vi "CAN FD.vi"() -> ()   [LabVIEW 2018]
uses:
  <vilib>/xnet/xnet.llb/XNET Create Session (Signal Input Single-point).vi
  <vilib>/xnet/xnet.llb/XNET Read (Signal Single-point).vi
  <resource>/objmgr/xnet.rc
panel:
  out "CAN:FD ISO Mode":u32(ring) items=["ISO", "Non ISO", "ISO Legacy"]
  out "PDUs Required?":bool
  out "element":refnum<k21>
  in  "stop":bool
  out "data":dbl[](array[numeric]) format="%.2f"
  out "session out 2":refnum<k21>
  out "Signals":refnum<k21>[](array[refnum])
  in  "error in (no error)":errorcluster
  in  "DBC File Selection":refnum<k21>="CAN DATA"
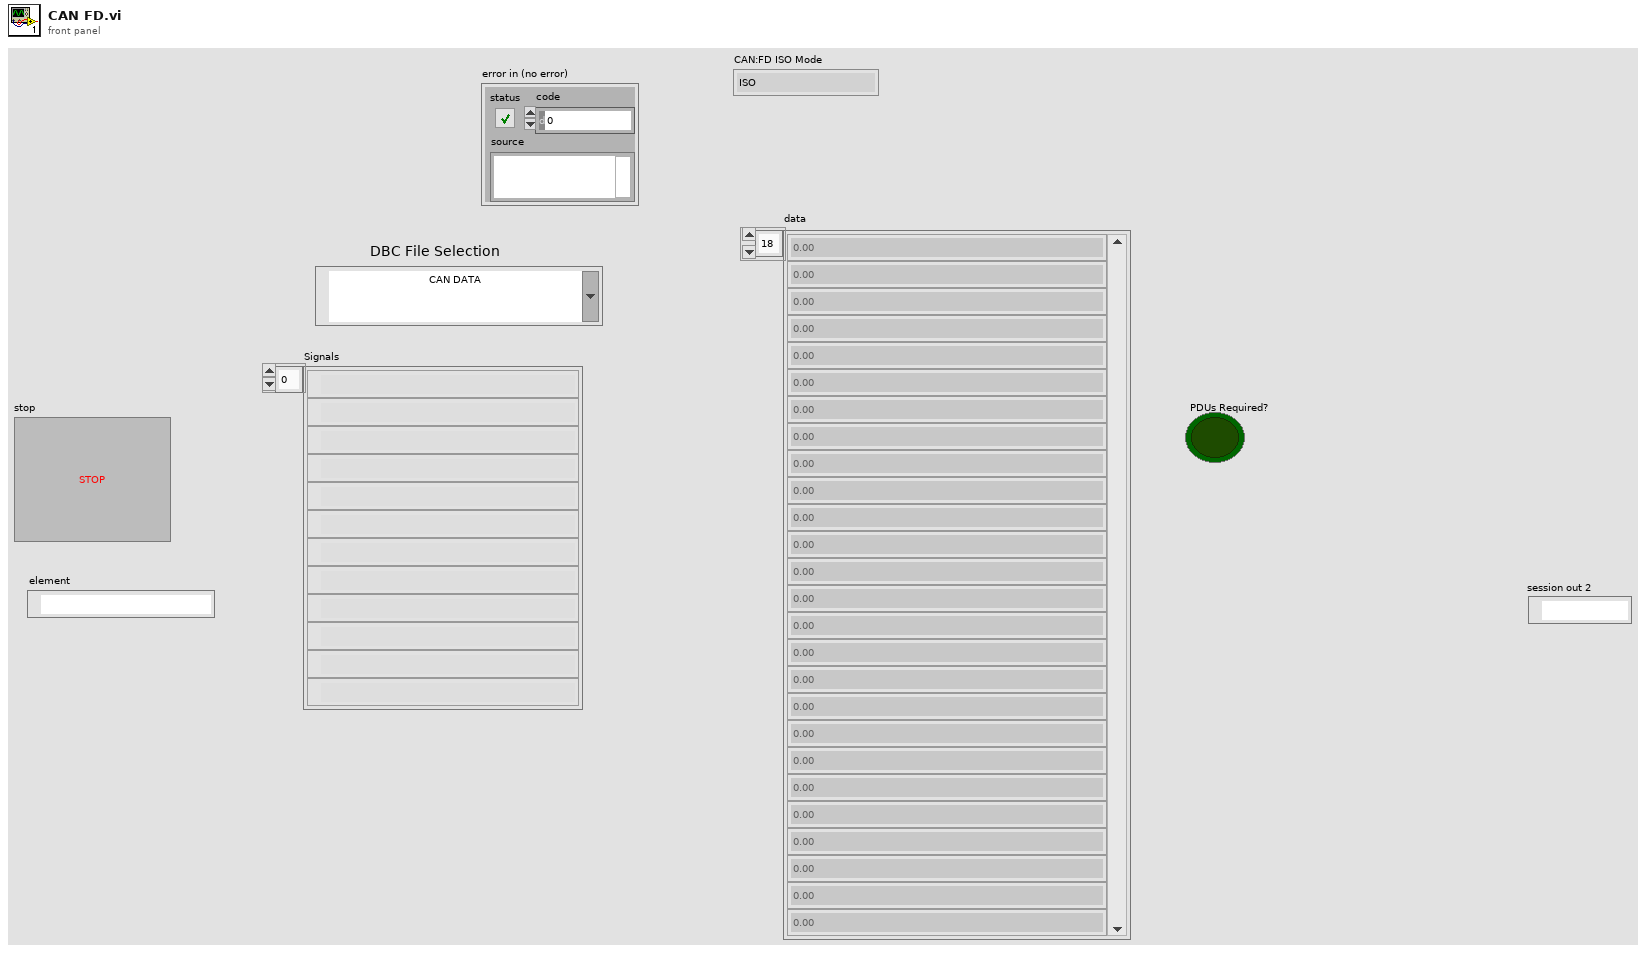
[diagram p1: front panel]
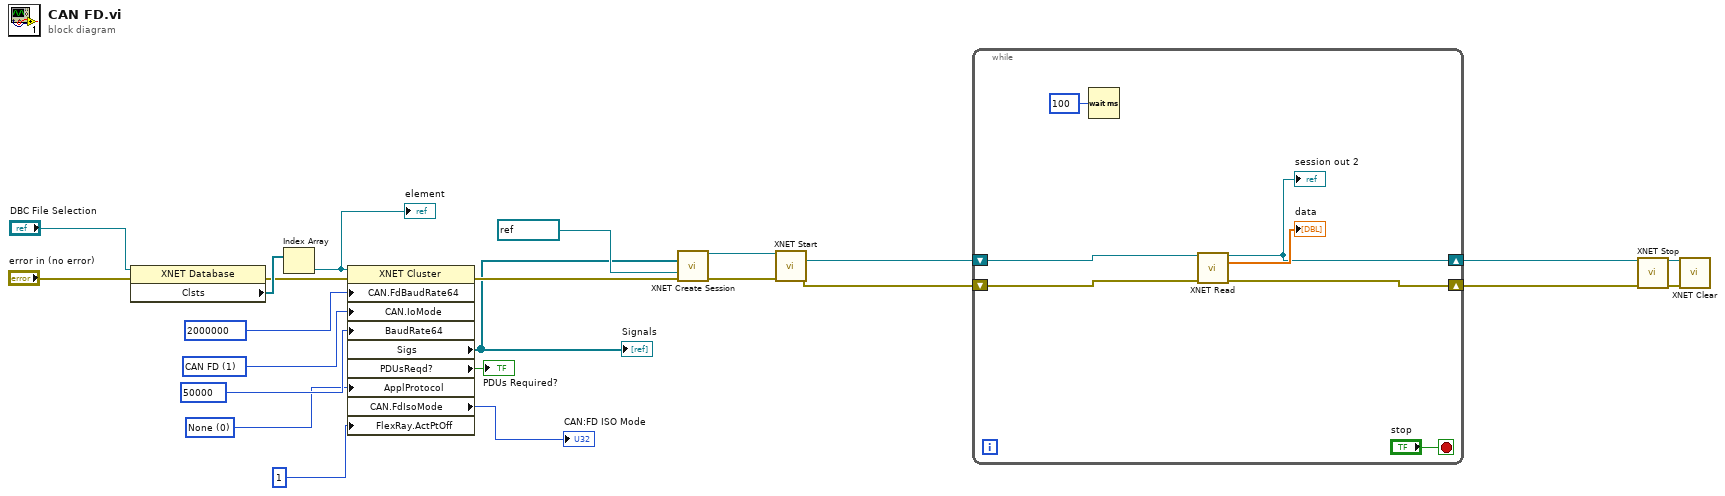
[diagram p0: block diagram]
diagram:
  w4 = u32 0 items=["None", "J1939"] ("Application Protocol")
  w19 = u32 1 items=["CAN 2.0", "CAN FD", "CAN FD+BRS"] ("CAN:I/O Mode")
  n1 = property class="XNET Database"(reference="DBC File Selection", error in="error in (no error)") -> (error out=w17:errorcluster, "Clsts"=w23:refnum<k21>[])  [unwired: 1 out]
  n2 = Index Array(array=w23) -> (element=w1:refnum<k21>)  [unwired: 1 in]
  "element" <- w1
  n3 = property class="XNET Cluster"(reference=w1, error in=w17, "CAN.FdBaudRate64"=u64 2000000 ("CAN:64bit FD Baud Rate"), "CAN.IoMode"=w19, "BaudRate64"=u64 50000 ("64bit Baud Rate"), "ApplProtocol"=w4, "FlexRay.ActPtOff"=u32 1 ("FlexRay:Action Point Offset")) -> (error out=w15:errorcluster, "Sigs"=w6:refnum<k21>[], "PDUsReqd?"=→"PDUs Required?":bool, "CAN.FdIsoMode"=→"CAN:FD ISO Mode":u32)  [unwired: 1 out]
  "Signals" <- w6
  n4 = call-poly <vilib>:"XNET Create Session.vi"("signal list"=w6, "interface"=refnum<k21> "CAN1" ("Select Interface"), "error in (no error)"=w15) -> ("session out"=w12:refnum<k21>, "error out"=w11:errorcluster)  [unwired: 11 out]
  n5 = call <vilib>:"XNET Start.vi"("session in"=w12, "error in (no error)"=w11) -> ("session out"=w13:refnum<k21>, "error out"=w14:errorcluster)  [unwired: 12 in]
  n6 = while {
    shift-right: [w26] -> w7
    shift-left: w14 -> [w29]
    shift-right: [w27] -> w8
    shift-left: w13 -> [w28]
    stop <- "stop" stop-if-true
    n7 = Wait (ms)(milliseconds to wait=u32 100) -> ()  [unwired: 1 out]
    n8 = call-poly <vilib>:"XNET Read.vi"("session in"=w28, "error in (no error)"=w29) -> ("session out"=w27:refnum<k21>, "data"=→"data":dbl[], "error out"=w26:errorcluster)  [unwired: 11 in]
    "session out 2" <- w27
  }
  n9 = call <vilib>:"XNET Stop.vi"("session in"=w8, "error in (no error)"=w7) -> ("session out"=w9:refnum<k21>, "error out"=w10:errorcluster)  [unwired: 12 in]
  n10 = call <vilib>:"XNET Clear.vi"("session in"=w9, "error in (no error)"=w10) -> ()  [unwired: 13 in, 1 out]
